vi "PLC_Launcher.vi"(6 "OpenPanel":bool, 7 "Type":T1, 8 "error in (no error)":errorcluster, 9 "Debug":bool, 10 "Context":refnum<vi>, 11 "ModuleName":string) -> (0 "error out":errorcluster, 3 "PLC Enqueuer":refnum<class "Message Enqueuer.lvclass">)   [LabVIEW 2025, in "PLC_API.lvlib"]
uses:
  PLC_API.lvlib
  <vilib>/ActorFramework/Message Enqueuer/Message Enqueuer.lvclass
  PLC_Module/PLC_Module/PLC_Type.ctl
  PLC_Module/PLC_Module/PLC_Module.lvclass
  Msg.ctl
  PLC_Module/PLC_Module/PLC_Module.lvclass/PLC_Module.ctl
  Module/Module/Module Messages/CoreComm Msg/CoreComm Msg.lvclass/CoreComm Msg.ctl
  <vilib>/ActorFramework/Message Enqueuer/Message Enqueuer.lvclass/Message Enqueuer.ctl
  3bdc3695-5b46-4f3b-abde-a37778213517.vi
  PLC_Module/PLC_Module/Write Type.vi
  <vilib>/ActorFramework/Message Enqueuer/Enqueue.vi
  Module/Module/Module Messages/CoreComm Msg/CoreComm Msg.lvclass
  <vilib>/ActorFramework/Message Priority Queue/Priority Enqueue.vi
  <vilib>/ActorFramework/Actor/Actor.lvclass
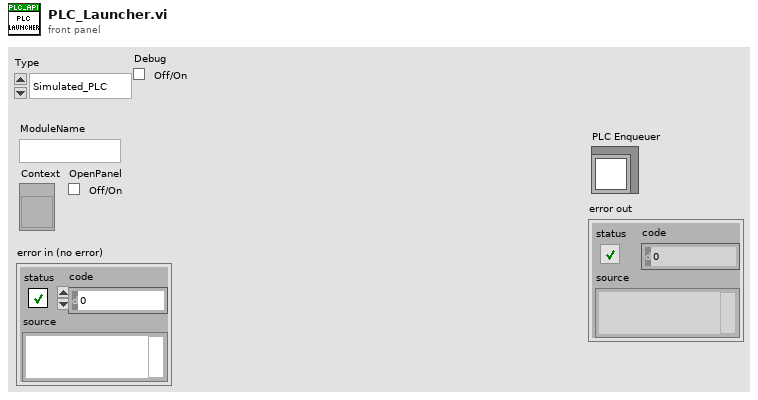
[diagram p1: front panel]
types:
  T1 = typedef "PLC_Module.lvlib/PLC_Module.lvclass/PLC_Type.ctl" = enum16{"Simulated_PLC", "SIMATIC_S7"}
  T2 = typedef "Msg.ctl" = string
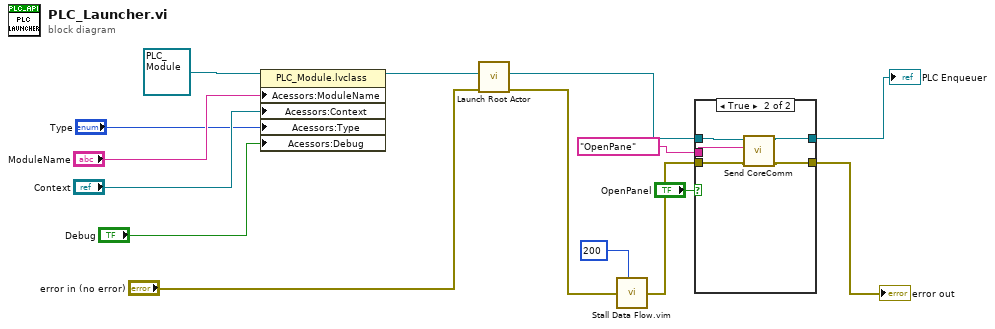
[diagram p0: block diagram]
diagram:
  n1 = property class="PLC_Module.lvclass"(reference=refnum<class "PLC_Module.lvclass"> refnum ("PLC_Module.lvlib:PLC_Module.lvclass"), "Acessors:ModuleName"="ModuleName", "Acessors:Context"="Context", "Acessors:Type"="Type", "Acessors:Debug"="Debug") -> (reference out=w13:refnum<class "PLC_Module.lvclass">)  [unwired: 1 in, 1 out]
  n2 = call <vilib>:"Launch Root Actor.vi"("error in (no error)"="error in (no error)", "Actor"=w13) -> ("error out"=w8:errorcluster, "Actor's Enqueuer"=w5:refnum<class "Message Enqueuer.lvclass">)  [unwired: 8 in]
  n3 = call "Stall Data Flow.vim"("value in"=w8, "milliseconds to wait"=u32 200) -> ("value out"=w4:errorcluster)  [unwired: 1 out]
  n4 = case shown="True" "OpenPanel" {
    tunnel: T2 "OpenPane" ("Msg") -> [_ w18]
    tunnel: w5 -> [w17 w22]
    tunnel: w4 -> [w16 w19]
    tunnel: [w16 w20] -> w3
    tunnel: [w17 w21] -> w2
    frame False {
    }
    frame True {
      n5 = call "Send CoreComm.vi"("error in (no error)"=w19, "Msg"=w18, "Message Enqueuer"=w22) -> ("error out"=w20:errorcluster, "Message Enqueuer out"=w21:refnum<class "Message Enqueuer.lvclass">)  [unwired: 7 in]
    }
  }
  "PLC Enqueuer" <- w2
  "error out" <- w3
